vi "FPGA_Set Digital Output.vi"(11 "Digital Output In":T1={"DO 0"="RMC/DIO62", "DO 1"="RMC/DIO44", "DO 2"="RMC/DIO77", "DO 3"="RMC/DIO61", "DO 4"="RMC/DIO94", "DO 5"="RMC/DIO12", "DO 6"="RMC/DIO76", "DO 7"="RMC/DIO29", "DO 8"="RMC/DIO93", "DO 9"="RMC/DIO11", "DO 10"="RMC/DIO43", "DO 11"="RMC/DIO28"}) -> (3 "Digital Output Out":T1={"DO 0"="RMC/DIO62", "DO 1"="RMC/DIO44", "DO 2"="RMC/DIO77", "DO 3"="RMC/DIO61", "DO 4"="RMC/DIO94", "DO 5"="RMC/DIO12", "DO 6"="RMC/DIO76", "DO 7"="RMC/DIO29", "DO 8"="RMC/DIO93", "DO 9"="RMC/DIO11", "DO 10"="RMC/DIO43", "DO 11"="RMC/DIO28"})   [LabVIEW 2018]
uses:
  Data Def/FPGA_Digital Output.ctl
  <vilib>/rvi/eio/common/nirviEmuTemplateMethod_errors.vi
  <vilib>/eio/EIOMethodNode/EIOMethodNode.xnode
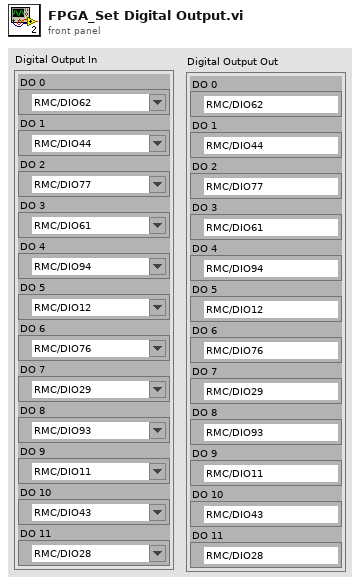
[diagram p1: front panel]
types:
  T1 = typedef "FPGA_Digital Output.ctl" = cluster{"DO 0":refnum<k21>, "DO 1":refnum<k21>, "DO 2":refnum<k21>, "DO 3":refnum<k21>, "DO 4":refnum<k21>, "DO 5":refnum<k21>, "DO 6":refnum<k21>, "DO 7":refnum<k21>, "DO 8":refnum<k21>, "DO 9":refnum<k21>, "DO 10":refnum<k21>, "DO 11":refnum<k21>}
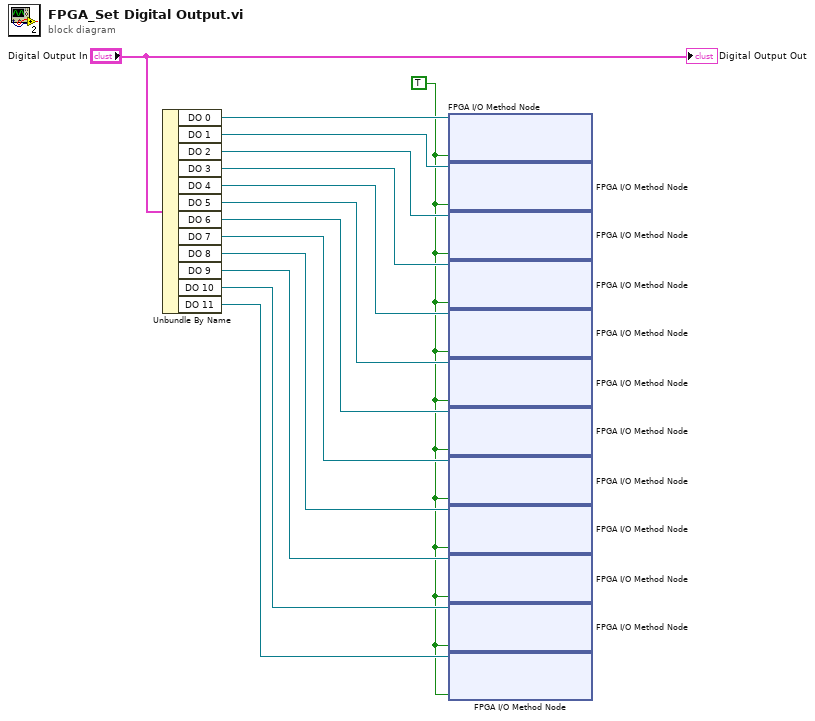
[diagram p0: block diagram]
diagram:
  w1 = TRUE ("Enable")
  n1 = Unbundle By Name("Digital Output In") -> ("DO 0"=w13:refnum<k21>, "DO 1"=w12:refnum<k21>, "DO 2"=w11:refnum<k21>, "DO 3"=w10:refnum<k21>, "DO 4"=w9:refnum<k21>, "DO 5"=w8:refnum<k21>, "DO 6"=w7:refnum<k21>, "DO 7"=w6:refnum<k21>, "DO 8"=w5:refnum<k21>, "DO 9"=w4:refnum<k21>, "DO 10"=w3:refnum<k21>, "DO 11"=w2:refnum<k21>)
  n2 = xnode "FPGA I/O Method Node"("FPGA I/O In"=w13, "Enable"=w1) -> ()  [unwired: 1 out]
  n3 = xnode "FPGA I/O Method Node"("FPGA I/O In"=w12, "Enable"=w1) -> ()  [unwired: 1 out]
  n4 = xnode "FPGA I/O Method Node"("FPGA I/O In"=w11, "Enable"=w1) -> ()  [unwired: 1 out]
  n5 = xnode "FPGA I/O Method Node"("FPGA I/O In"=w10, "Enable"=w1) -> ()  [unwired: 1 out]
  n6 = xnode "FPGA I/O Method Node"("FPGA I/O In"=w9, "Enable"=w1) -> ()  [unwired: 1 out]
  n7 = xnode "FPGA I/O Method Node"("FPGA I/O In"=w8, "Enable"=w1) -> ()  [unwired: 1 out]
  n8 = xnode "FPGA I/O Method Node"("FPGA I/O In"=w7, "Enable"=w1) -> ()  [unwired: 1 out]
  n9 = xnode "FPGA I/O Method Node"("FPGA I/O In"=w6, "Enable"=w1) -> ()  [unwired: 1 out]
  n10 = xnode "FPGA I/O Method Node"("FPGA I/O In"=w5, "Enable"=w1) -> ()  [unwired: 1 out]
  n11 = xnode "FPGA I/O Method Node"("FPGA I/O In"=w4, "Enable"=w1) -> ()  [unwired: 1 out]
  n12 = xnode "FPGA I/O Method Node"("FPGA I/O In"=w3, "Enable"=w1) -> ()  [unwired: 1 out]
  n13 = xnode "FPGA I/O Method Node"("FPGA I/O In"=w2, "Enable"=w1) -> ()  [unwired: 1 out]
  "Digital Output Out" <- "Digital Output In"
